vi "IIR Cascade Filter with I.C. (CDB).vi"(3 "Initial Filter State":cdb[](array[numeric]), 4 "IIR Filter Cluster":T1 {"Forward Coefficients" format="%.4f"; "Reverse Coefficients" format="%.4f"}, 5 "X":cdb[](array[numeric])) -> (0 "error":i32, 1 "Final Filter State":cdb[](array[numeric]), 2 "Filtered X":cdb[](array[numeric]))   [LabVIEW 2018, in "NI_AALBase.lvlib"]
doc: "Filters the input sequence <B>X</B> using the cascade form of the IIR filter specified by the <B>IIR Filter Cluster</B>. This VI is similar to the IIR Cascade Filter VI except that you specify the initial conditions for this VI. Wire data to the <B>X</B> input to determine the polymorphic instance to use or manually select the instance."
uses:
  NI_AALBase.lvlib
  <resource>/lvanlys.dll
panel:
  # "IIR Cascade Filter\n with I.C."
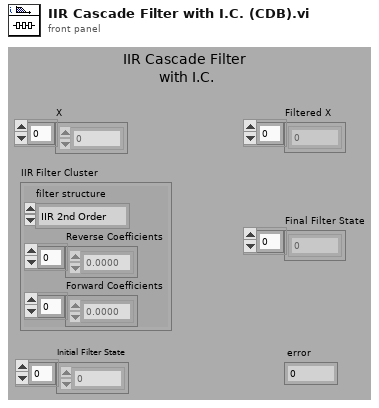
[diagram p1: front panel]
types:
  T1 = cluster{"filter structure":enum32{"IIR 2nd Order", "IIR 4th Order"}, "Reverse Coefficients":dbl[], "Forward Coefficients":dbl[]}
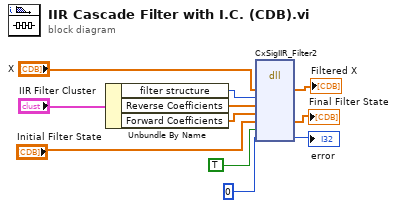
[diagram p0: block diagram]
diagram:
  n1 = Unbundle By Name("IIR Filter Cluster") -> ("filter structure"=w6:enum32{"IIR 2nd Order", "IIR 4th Order"}, "Reverse Coefficients"=w10:dbl[], "Forward Coefficients"=w11:dbl[])
  n2 = dll-call lib="C:/Program Files (x86)/National Instruments/LabVIEW 2018/resource/lvanlys.*" fn="CxSigIIR_Filter2"("X"="X", "filter structure"=w6, "aH"=w10, "bH"=w11, "Initial Filter State"="Initial Filter State", "output param"=TRUE, "output param"=0) -> ("X"=→"Filtered X":cdb[], "Initial Filter State"=→"Final Filter State":cdb[], "output param"=→"error":i32)  [unwired: 8 in, 2 out]
